vi "GFV_LoggingQueue.vi"(7 "GFV Action":T1, 8 "error in (no error)":errorcluster, 11 "Message queue in":refnum<queue>) -> (0 "error out":errorcluster, 3 "Message queue out":refnum<queue>)   [LabVIEW 2015]
doc: "Global Functional Variable (GFV) containing the queue used to return logging messages from the library.\n\nNote: Deleting the queue reference does not close it, use relase queue after deleting."
uses:
  Controls/GFV Action.ctl
  Controls/LOG_MessageQueue.ctl
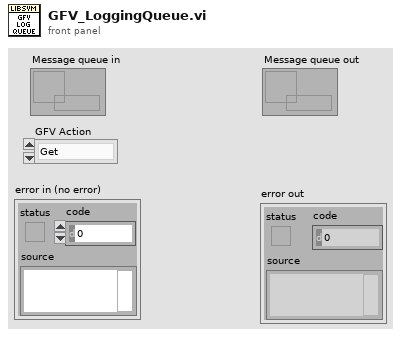
[diagram p1: front panel]
types:
  T1 = typedef "GFV Action.ctl" = enum16{"Get", "Set", "Delete"}
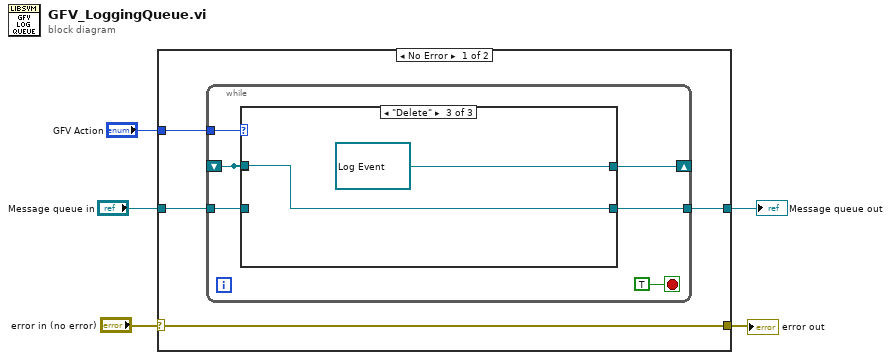
[diagram p0: block diagram]
diagram:
  n1 = case shown="No Error" "error in (no error)" {
    selector: "error in (no error)" -> [w8 w21]
    tunnel: [w8 w21] -> w5
    tunnel: "GFV Action" -> [w9 _]
    tunnel: "Message queue in" -> [w7 w20]
    tunnel: [w6 w20] -> w1
    frame No Error {
      n2 = while {
        tunnel: w9 -> [w14]
        tunnel: w7 -> [w13]
        shift-right: [w12] -> _
        shift-left: _ -> [w10]
        tunnel: [w11] -> w6
        stop <- TRUE stop-if-true
        n3 = case shown="\"Delete\"" w14 {
          tunnel: w13 -> [_ w17 _]
          tunnel: [w16 w17 refnum<queue> refnum ("Message queue in")] -> w12
          tunnel: [w16 w17 w18] -> w11
          tunnel: w10 -> [w16 _ _]
          tunnel: w10 -> [_ _ w18]
          frame "Get", Default {
          }
          frame "Set" {
          }
          frame "Delete" {
          }
        }
      }
    }
    frame Error {
    }
  }
  "error out" <- w5
  "Message queue out" <- w1
